vi "Game_returnFinalNotif.vi"(8 "error in (no error)":errorcluster, 11 "notifier":refnum<notifier>) -> (0 "error out":errorcluster)   [LabVIEW 2020]
uses:
  Typedefs/communicationData.ctl
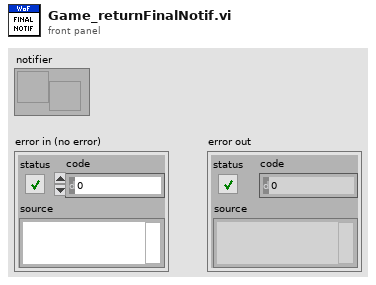
[diagram p1: front panel]
types:
  T1 = typedef "communicationData.ctl" = cluster{"command":string, "payload":variant, "response":variant}
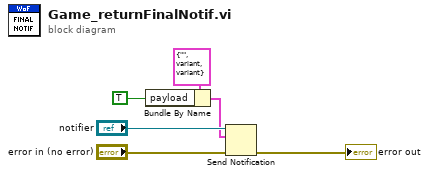
[diagram p0: block diagram]
diagram:
  n1 = Bundle By Name(cluster=T1 {"command"="", "payload"=variant, "response"=variant} ("communication"), "payload"=TRUE) -> (w2:T1)
  n2 = Send Notification(notification=w2, notifier="notifier", error in (no error)="error in (no error)") -> (error out=→"error out":errorcluster)  [unwired: 1 out]
